vi "fluorescence.vi"() -> ()   [LabVIEW 2012]
uses:
  <vilib>/Utility/file.llb/Write To Spreadsheet File (DBL).vi
panel:
  in  "time Step":dbl=5.0
  out "CurrentWaveForm":digitalwaveform(waveform)={"t0"=timestamp(0 s since 1904-01-01), "dt"=1e-07, "Y"={"transitions"=[0, 2100, 2200, 2300, 2301, 2311, 2361, 2461], "data"=[[1, 1, 1, 0, 0], [1, 0, 1, 0, 0], [1, 0, 0, 0, 0], [0, 0, 0, 0, 0], [0, 0, 0, 0, 0], [0, 0, 0, 0, 1], [0, 0, 0, 0, 0], [0, 1, 1, 0, 0]]}, "error"={"status"=FALSE, "code"=37421928, "source"=""}}
  out "binned path":path=path "c:/data/1762 Scans/2016-09-26-scans/2016-09-26_15-23-04_1762scanWithPumping.txt"
  out "Path":path=path "c:/data/1762 Scans/2016-09-26_15-23-04_1762scanWithPumping.txt"
  in  "PMT Sample Time":dbl=0.05 format="%0.2f"
  in  "Stop Scan":bool
  in  "Delete Data":bool
  out "ExptWvfm":digitalwaveform(waveform)={"t0"=timestamp(0 s since 1904-01-01), "dt"=1e-07, "Y"={"transitions"=[0, 2100, 2200, 2300, 2301, 2411], "data"=[[1, 1, 1, 0, 0], [1, 0, 1, 0, 0], [1, 0, 0, 0, 0], [0, 0, 0, 0, 0], [0, 0, 0, 0, 0], [0, 1, 1, 0, 0]]}, "error"={"status"=FALSE, "code"=37421928, "source"=""}}
  out "PMT Counts":i32(graph)=1168
  out "Counts after 1762":i32=1168
  out "OuterLoop":i32
  out "InnerLoop":i32
  out "Bright Events":dbl
  in  "Discriminator Level\n (Bright/Dark)":i32=100
  out "digital waveform out 2":digitalwaveform(waveform)={"t0"=timestamp(0 s since 1904-01-01), "dt"=1e-07, "Y"={"transitions"=[0, 2100, 2200, 2300, 2301, 2411], "data"=[[1, 1, 1, 0, 0], [1, 0, 1, 0, 0], [1, 0, 0, 0, 0], [0, 0, 0, 0, 0], [0, 0, 0, 0, 0], [0, 1, 1, 0, 0]]}, "error"={"status"=FALSE, "code"=37421928, "source"=""}}
  in  "1762 frequency":dbl=84.24
  in  "Comment":string=" "
  in  "B Field":dbl=999.0
  in  "RF Power":dbl=999.0
  in  "Runs per data point":dbl=50.0
  in  "Stop Time":dbl(slide)=100.0 min=0.0 max=5000.0 step=1.0 scale=0.0..100.0 scale format="%#.5f"
  in  "Start Time":dbl(slide) min=0.0 max=1000.0 step=1.0 scale=0.0..100.0 scale format="%#.0f"
  out "Cur Time":dbl format="%#_8f"
  out "Frequency Scan":cluster{dbl, dbl}[](graph)=[{85300000.0, 1.0}, {85290000.0, 1.0}, {85280000.0, 1.0}, {85270000.0, 1.0}, {85260000.0, 1.0}, {85250000.0, 1.0}, {85240000.0, 1.0}, {85230000.0, 1.0}, {85220000.0, 1.0}, {85210000.0, 1.0}, {85200000.0, 1.0}, {85190000.0, 1.0}, {85180000.0, 1.0}, {85170000.0, 1.0}, {85160000.0, 1.0}, {85150000.0, 1.0}, {85140000.0, 1.0}, {85130000.0, 1.0}, {85120000.0, 1.0}, {85110000.0, 1.0}, {85100000.0, 1.0}, {85090000.0, 1.0}, {85080000.0, 1.0}, {85070000.0, 1.0}, {85060000.0, 1.0}, {85050000.0, 1.0}, {85040000.0, 1.0}, {85030000.0, 1.0}, {85020000.0, 1.0}, {85010000.0, 1.0}, {85000000.0, 1.0}, {84990000.0, 1.0}, {84980000.0, 1.0}, {84970000.0, 1.0}, {84960000.0, 1.0}, {84950000.0, 1.0}, {84940000.0, 1.0}, {84930000.0, 1.0}, {84920000.0, 1.0}, {84910000.0, 1.0}, {84900000.0, 1.0}]
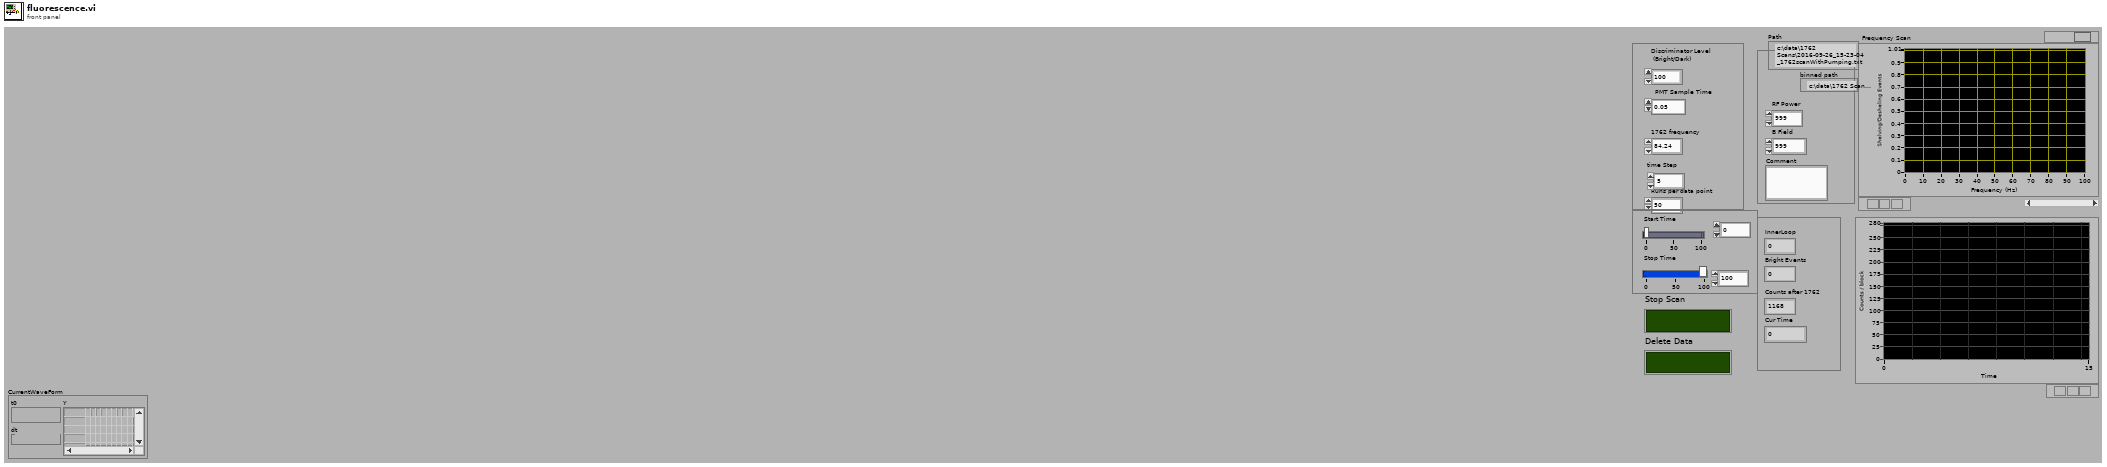
[diagram p1: front panel]
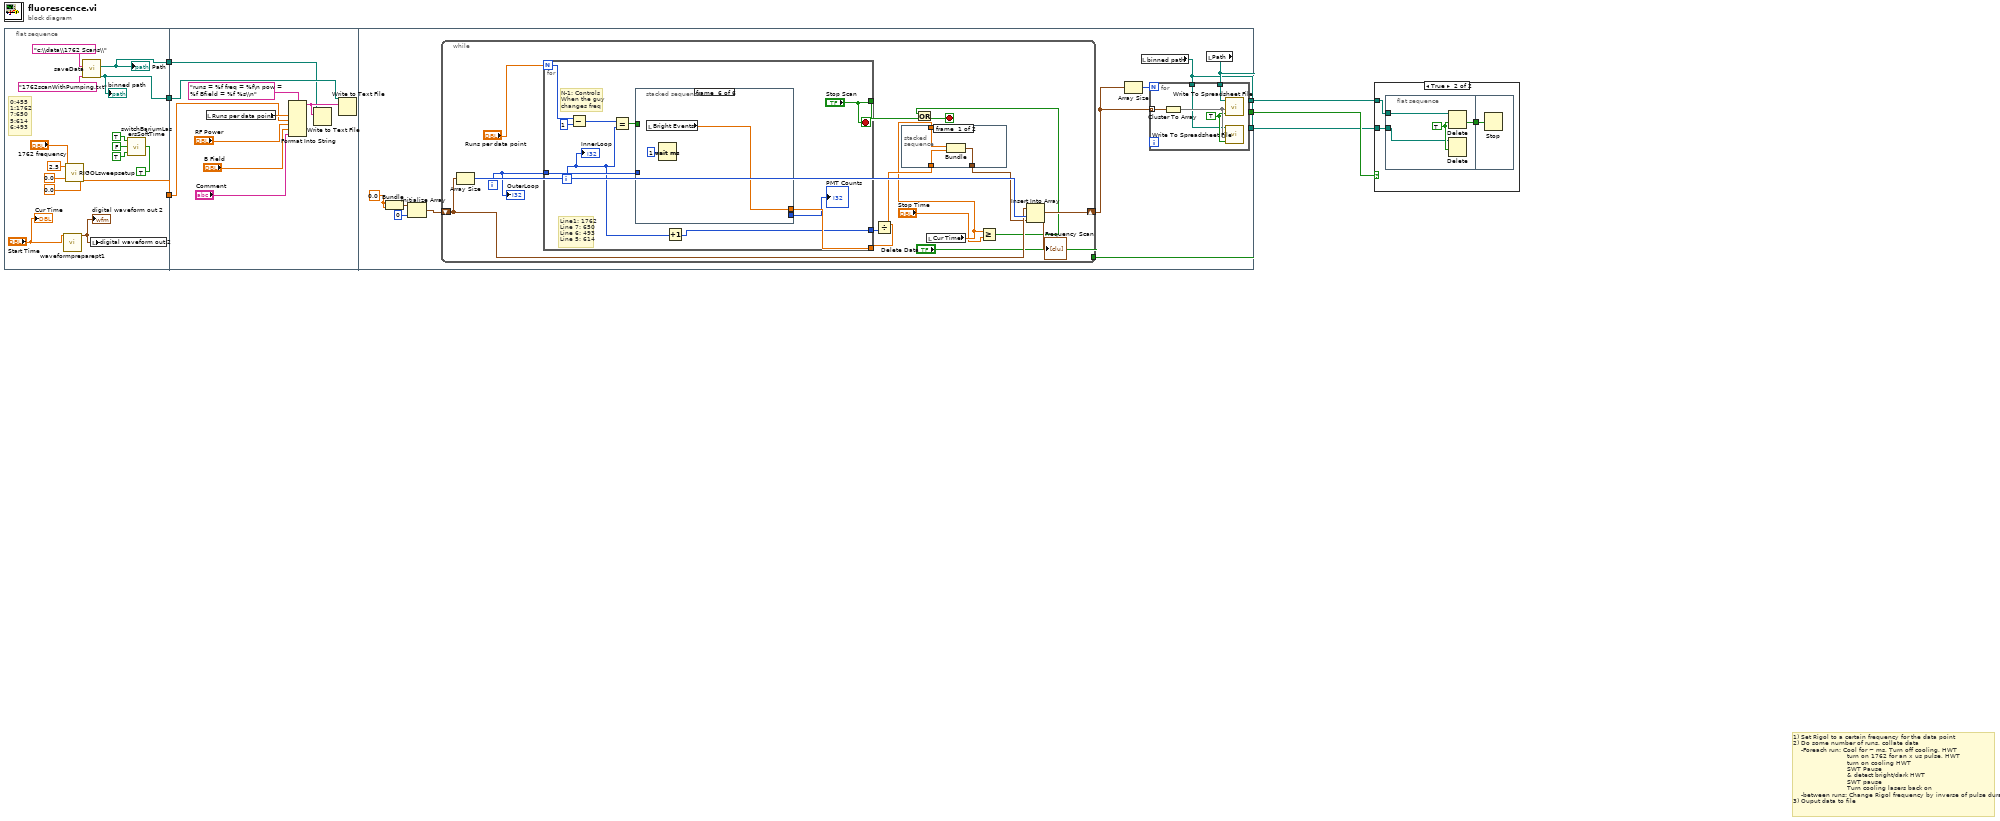
[diagram p0: block diagram]
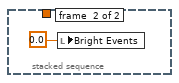
[diagram p3: hidden frame]
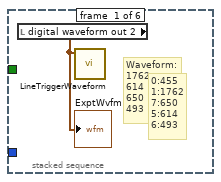
[diagram p4: hidden frame]
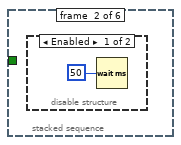
[diagram p5: hidden frame]
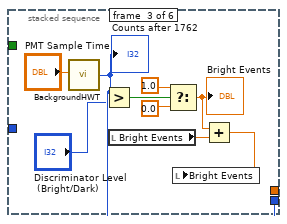
[diagram p7: hidden frame]
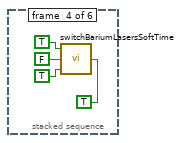
[diagram p8: hidden frame]
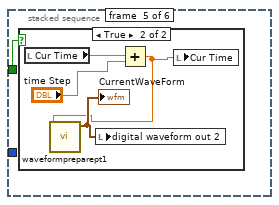
[diagram p9: hidden frame]
diagram:
  # "1) Set Rigol to a certain frequency for the data point\n2) Do some number of runs, collate data\n    -Foreach run: Cool for ~ ms, Turn off cooling, HWT\n                           turn on 1762 for an x us pulse, HWT\n                           turn on cooling HWT\n                           SWT Pause\n                           & detect bright/dark HWT\n                           SWT pause\n                           Turn cooling lasers back on \n    -between runs: Change Rigol frequency by inverse of pulse duration\n3) Ouput data to file"
  n1 = flat-sequence {
    tunnel: [w19] -> w6
    tunnel: [w16] -> w5
    tunnel: ["1762 frequency"] -> w1
    tunnel: w6 -> [w29]
    tunnel: w5 -> [w22]
    tunnel: w1 -> [w21]
    tunnel: [w32] -> w4
    tunnel: [w31] -> w3
    tunnel: [w30] -> w2
    frame #0 {
      # "0:455\n1:1762\n7:650\n5:614\n6:493"
      n2 = call "waveformpreparept1.vi"("1762 pulse length (units of 1 us)"="Start Time") -> ("digital waveform out 2"=w20:digitalwaveform)  [unwired: 8 in]
      "digital waveform out 2" <- w20
      n3 = call "RIGOLsweepsetup.vi"("AP Sweep Width (MHz)"=0.0, "Time (ms)"=0.0, "Amplitude (Vpp)"=2.5, "Frequency (MHz)"="1762 frequency") -> ()  [unwired: 8 in]
      n4 = call "saveData.vi"("filename"="1762scanWithPumping.txt", "dataDirectory"="c:\\data\\1762 Scans\\") -> ("binned path"=w19:path, "Path"=w16:path)  [unwired: 8 in]
      "Path" <- w16
      "binned path" <- w19
      n5 = local write "digital waveform out 2"(w20) -> ()
      n6 = call "switchBariumLasersSoftTime.vi"("650"=TRUE, "614"=TRUE, "1762"=FALSE, "493"=TRUE) -> ()  [unwired: 2 in]
      "Cur Time" <- "Start Time"
    }
    frame #1 {
      n7 = local read "Runs per data point"() -> (w27:dbl)
      n8 = Format Into String(format string="runs = %f freq = %f\n pow = %f Bfield = %f %s\\n", w27, w21, "RF Power", "B Field", "Comment") -> (resulting string=w23:string)  [unwired: 2 in, 1 out]
      n9 = Write to Text File(file (use dialog)=w22, text=w23) -> ()  [unwired: 2 in, 3 out]
      n10 = Write to Text File(file (use dialog)=w29, text=w23) -> ()  [unwired: 2 in, 3 out]
    }
    frame #2 {
      w37 = 0.0
      n11 = Bundle(w37, w37) -> (w38:cluster{dbl, dbl})  [unwired: 1 in]
      n12 = Initialize Array(w38, 0) -> (w35:cluster{dbl, dbl}[])
      n13 = while {
        shift-right: [w56] -> w33
        shift-left: w35 -> [w57]
        tunnel: ["Delete Data"] -> w32
        i -> [w55]
        stop <- w48 stop-if-true
        n14 = Array Size(array=w57) -> (size(s)=w58:i32)
        n15 = for {
          N: "Runs per data point" -> [w69]
          tunnel: [w68] -> w53
          tunnel: w55 -> [w67]
          tunnel: ["Stop Scan"] -> w50
          tunnel: [w63] -> w44
          i -> [w64]
          stop <- "Stop Scan" stop-if-true
          # "Line1: 1762\nLine 7: 650\nLine 6: 493\nLine 5: 614"
          # "N-1: Controls\nWhen the guy\nchanges freq"
          n16 = Subtract(x=w69, y=1) -> (x-y=w72:i32)
          n17 = Equal?(x=w72, y=w64) -> (x = y?=w70:bool)
          n18 = stacked-sequence {
            tunnel: w67 -> [_ _ _ _ _ _]
            tunnel: [_ _ w78 _ _ _] -> w66
            tunnel: w70 -> [_ _ _ _ w88 _]
            tunnel: [_ _ _ _ _ w93] -> w68
            frame #0 {
              # "0:455\n1:1762\n7:650\n5:614\n6:493"
              # "Waveform:\n1762\n614\n650\n493"
              n19 = local read "digital waveform out 2"() -> (w73:digitalwaveform)
              "ExptWvfm" <- w73
              n20 = call "LineTriggerWaveform.vi"("digital waveform in"=w73) -> ()  [unwired: 11 in]
            }
            frame #1 {
              n21 = disable-structure shown="Enabled" {
                frame Enabled {
                  n22 = Wait (ms)(milliseconds to wait=u32 50) -> ()  [unwired: 1 out]
                }
                frame Disabled {
                }
              }
            }
            frame #2 {
              n23 = call "BackgroundHWT.vi"("Sample Time(seconds)"="PMT Sample Time") -> ("Counts"=w78:i32)
              "Counts after 1762" <- w78
              n24 = Greater?(x=w78, y="Discriminator Level\n (Bright/Dark)") -> (0:w76:bool)
              n25 = local read "Bright Events"() -> (w79:dbl)
              n26 = Select(t=1.0, s=w76, f=0.0) -> (s? t:f=w81:dbl)
              "Bright Events" <- w81
              n27 = Add(x=w81, y=w79) -> (x+y=w80:dbl)
              n28 = local write "Bright Events"(w80) -> ()
            }
            frame #3 {
              n29 = call "switchBariumLasersSoftTime.vi"("650"=TRUE, "614"=TRUE, "1762"=FALSE, "493"=TRUE) -> ()  [unwired: 2 in]
            }
            frame #4 {
              n30 = case shown="True" w88 {
                frame False {
                }
                frame True {
                  n31 = local read "Cur Time"() -> (w91:dbl)
                  n32 = Add(x=w91, y="time Step") -> (x+y=w89:dbl)
                  n33 = call "waveformpreparept1.vi"("1762 pulse length (units of 1 us)"=w89) -> ("digital waveform out 2"=w92:digitalwaveform)  [unwired: 8 in]
                  "CurrentWaveForm" <- w92
                  n34 = local write "digital waveform out 2"(w92) -> ()
                  n35 = local write "Cur Time"(w89) -> ()
                }
              }
            }
            frame #5 {
              n36 = local read "Bright Events"() -> (w93:dbl)
              n37 = Wait (ms)(milliseconds to wait=u32 1) -> ()  [unwired: 1 out]
            }
          }
          "PMT Counts" <- w66
          n38 = Increment(x=w64) -> (x+1=w63:i32)
          "InnerLoop" <- w64
        }
        n39 = Divide(x=w53, y=w44) -> (x/y=w52:dbl)
        n40 = local read "Cur Time"() -> (w46:dbl)
        n41 = stacked-sequence {
          tunnel: w52 -> [w61 _]
          tunnel: [w60 _] -> w54
          tunnel: w46 -> [w59 _]
          frame #0 {
            n42 = Bundle("Cur Time"=w59, w61) -> (w60:cluster{"Cur Time":dbl, dbl})  [unwired: 1 in]
          }
          frame #1 {
            n43 = local write "Bright Events"(0.0 ("Bright Events")) -> ()
          }
        }
        n44 = Greater Or Equal?(x=w46, y="Stop Time") -> (x >= y?=w47:bool)
        n45 = Or(x=w47, y=w50) -> (x .or. y?=w48:bool)
        n46 = Insert Into Array(array=w57, index=w58, new element=w54) -> (w56:cluster{dbl, dbl}[])
        "Frequency Scan" <- w56
        "OuterLoop" <- w55
      }
      n47 = Array Size(array=w33) -> (size(s)=w34:i32)
      n48 = local read "binned path"() -> (w30:path)
      n49 = local read "Path"() -> (w31:path)
      n50 = for {
        N: w34 -> [_]
        tunnel: w33 -> [w43] mode=indexing
        tunnel: w30 -> [w40]
        tunnel: w31 -> [w39]
        w41 = TRUE
        n51 = Cluster To Array(cluster=w43) -> (array=w42:dbl[])
        n52 = call-poly <vilib>:"Write To Spreadsheet File.vi"("append to file? (new file:F)"=w41, "1D data"=w42, "file path (dialog if empty)"=w39) -> ()  [unwired: 5 in, 1 out]
        n53 = call-poly <vilib>:"Write To Spreadsheet File.vi"("append to file? (new file:F)"=w41, "1D data"=w42, "file path (dialog if empty)"=w40) -> ()  [unwired: 5 in, 1 out]
      }
    }
  }
  n54 = case shown="True" w4 {
    tunnel: w3 -> [_ w96]
    tunnel: w2 -> [_ w95]
    frame False {
    }
    frame True {
      n55 = flat-sequence {
        tunnel: [w101] -> w97
        tunnel: w96 -> [w99]
        tunnel: w95 -> [w98]
        tunnel: w97 -> [w102]
        frame #0 {
          w100 = TRUE ("confirm (F)")
          n56 = Delete(path (use dialog)=w99, confirm (F)=w100) -> (cancelled=w101:bool)  [unwired: 3 in, 2 out]
          n57 = Delete(path (use dialog)=w98, confirm (F)=w100) -> ()  [unwired: 3 in, 3 out]
        }
        frame #1 {
          n58 = Stop(stop? (T)=w102) -> ()
        }
      }
    }
  }
